vi "Add_Part_of_Track(After_101)-1.vi"(0 "[IN] Still connected\ntracks in group":T3, 1 "[IN] # of subtrack conta\nining problem point":i32, 2 "[IN] Index of problem\npoint inside subtrack":i32, 3 "[IN] Minimal Sub\ntrack Length":i32, 7 "[IN] Subtracks":T1(array[cluster]), 9 "[IN] Count of variants":i32, 11 "error IN":errorcluster, 12 "[IN] Subtrack":T2, 13 "[IN] Index in subtrack":i32) -> (8 "[OUT] Subtracks":T1(array[cluster]), 10 "[OUT] Count of variants":i32, 15 "error OUT":errorcluster)   [LabVIEW 2013]
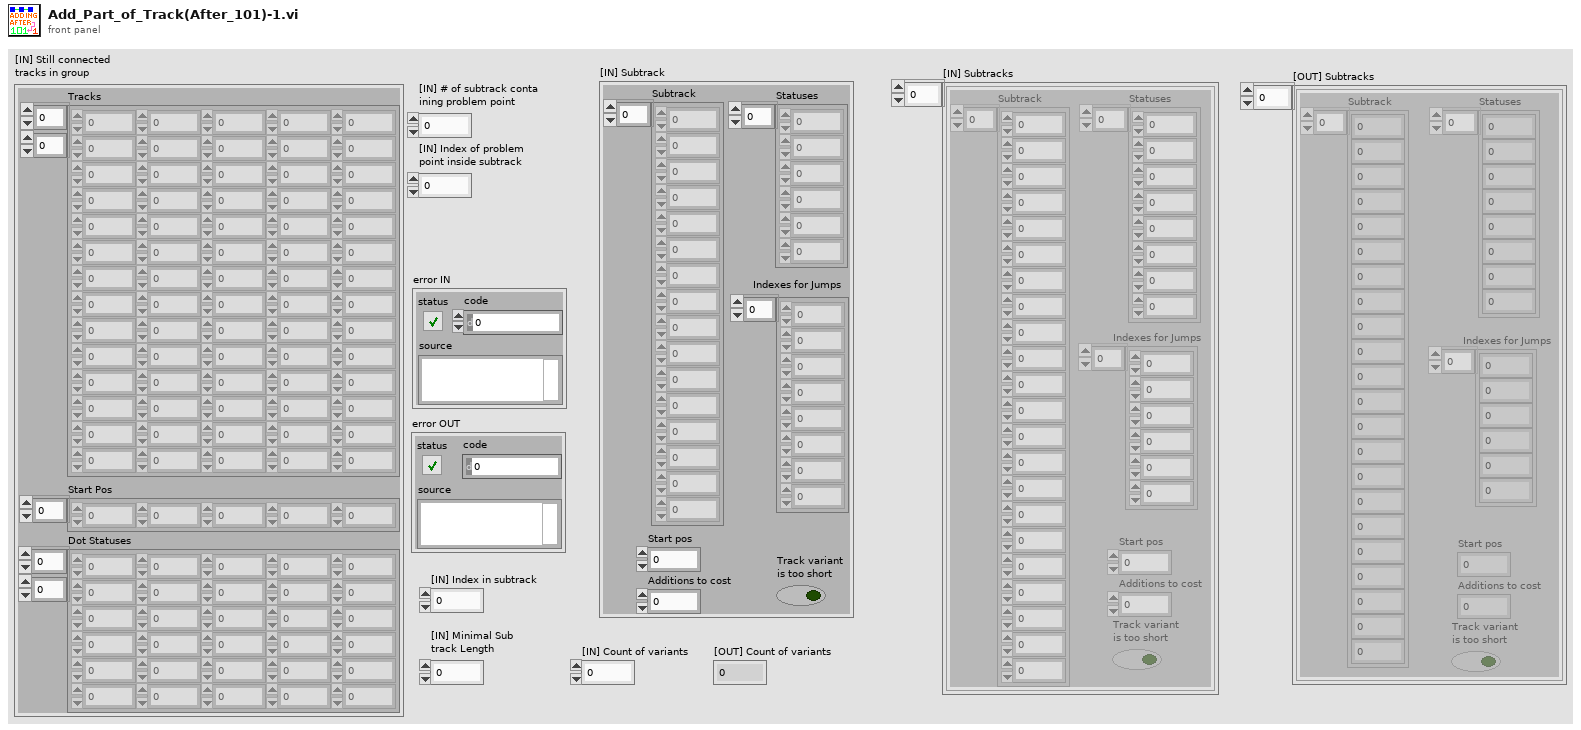
[diagram p1: front panel]
types:
  T1 = cluster{"Subtrack":dbl[], "Statuses":i16[], "Start pos":i32, "Additions to cost":i32, "Track variant \nis too short":bool, "Indexes for Jumps":i32[]}[]
  T2 = cluster{"Subtrack":dbl[], "Statuses":i16[], "Start pos":i32, "Additions to cost":i32, "Track variant \nis too short":bool, "Indexes for Jumps":i32[]}
  T3 = cluster{"Tracks":dbl[][], "Start Pos":i32[], "Dot Statuses":i16[][]}
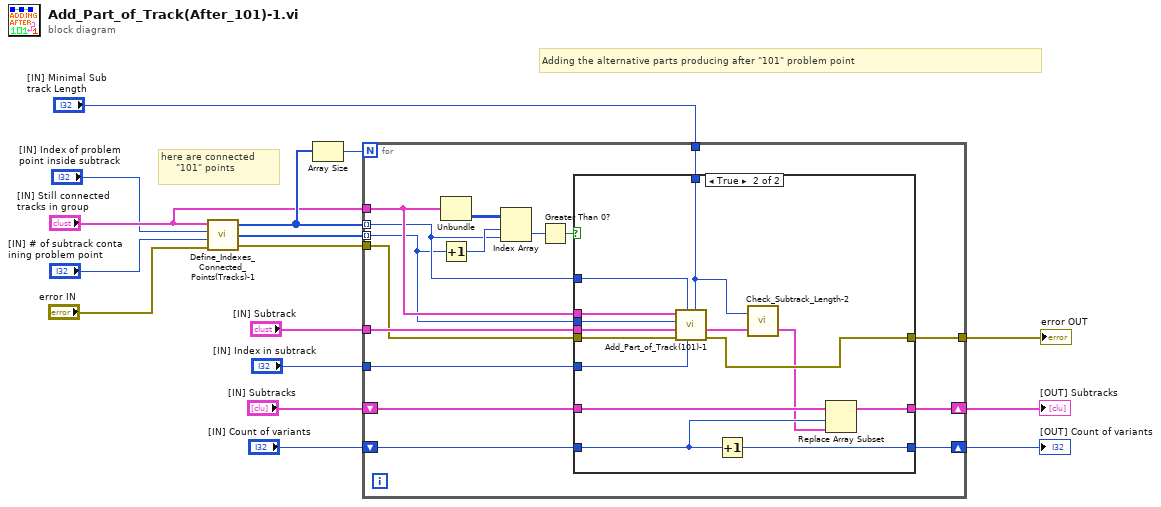
[diagram p0: block diagram]
diagram:
  # "here are connected \n     \"101\" points"
  # "Adding the alternative parts producing after \"101\" problem point"
  n1 = call "Define_Indexes_Connected_Points(Tracks)-1.vi"("error IN"="error IN", "[IN] Index of track with\n(problem displacement)"="[IN] # of subtrack conta\nining problem point", "[IN]Index of problem\ndisplacement inside track"="[IN] Index of problem\npoint inside subtrack", "[IN] Track group"="[IN] Still connected\ntracks in group") -> ("error OUT"=w13:errorcluster, "[OUT] Index of \nconnected dots\ninside the track"=w11:i32[], "[OUT] Index of connected\ntracks with problem dot"=w12:i32[])
  n2 = Array Size(array=w12) -> (size(s)=w14:i32)
  n3 = for {
    N: w14 -> [_]
    tunnel: w13 -> [w27]
    tunnel: w12 -> [w23] mode=indexing
    tunnel: w11 -> [w22] mode=indexing
    tunnel: "[IN] Still connected\ntracks in group" -> [w26]
    tunnel: "[IN] Subtrack" -> [w28]
    tunnel: "[IN] Index in subtrack" -> [w25]
    tunnel: "[IN] Minimal Sub\ntrack Length" -> [w24]
    shift-right: [w19] -> w2
    shift-left: "[IN] Subtracks" -> [w21]
    shift-right: [w18] -> w3
    shift-left: "[IN] Count of variants" -> [w20]
    tunnel: [w17] -> w1
    n4 = Unbundle(w26) -> ("Dot Statuses"=w30:i16[][])  [unwired: 2 out]
    n5 = Increment(x=w22) -> (x+1=w32:i32)
    n6 = Index Array(array=w30, index (row)=w32, index (col)=w23) -> (element=w31:i16)
    n7 = Greater Than 0?(x=w31) -> (x > 0?=w29:bool)
    n8 = case shown="True" w29 {
      tunnel: w28 -> [_ w49]
      tunnel: w27 -> [w33 w48]
      tunnel: w26 -> [_ w47]
      tunnel: w25 -> [_ w46]
      tunnel: w24 -> [_ w37]
      tunnel: w23 -> [_ w45]
      tunnel: w22 -> [_ w44]
      tunnel: w21 -> [w35 w43]
      tunnel: w20 -> [w34 w42]
      tunnel: [w34 w41] -> w18
      tunnel: [w35 w40] -> w19
      tunnel: [w33 w39] -> w17
      frame False {
      }
      frame True {
        n9 = call "Add_Part_of_Track(101)-1.vi"("[IN] Minimal Sub\ntrack Length"=w37, "[IN] Index in subtrack"=w46, "[IN] # of subtrack conta\nining problem point"=w45, "error IN"=w48, "[IN] Subtrack"=w49, "[IN] Index of problem\npoint inside subtrack"=w44, "[IN] Still connected\ntracks in group"=w47) -> ("error OUT"=w39:errorcluster, "[OUT] Subtrack"=w38:T2)  [unwired: 2 in, 1 out]
        n10 = Increment(x=w42) -> (x+1=w41:i32)
        n11 = call "Check_Subtrack_Length-2.vi"("[IN] Subtrack"=w38, "[IN] Minimal Sub\ntrack Length"=w37) -> ("[OUT] Subtrack"=w36:T2)  [unwired: 1 in]
        n12 = Replace Array Subset(array=w43, new element=w36, index=w42) -> (w40:T1)
      }
    }
  }
  "error OUT" <- w1
  "[OUT] Subtracks" <- w2
  "[OUT] Count of variants" <- w3
